vi "DSF.Shared.Constants.Library Name.Engine.vi"() -> (3 "Engine Library Name":string)   [LabVIEW 2017, in "DSF.Engine.lvlib"]
uses:
  DSF.Engine.lvlib
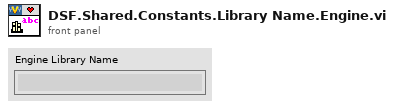
[diagram p1: front panel]
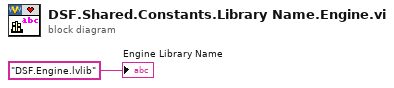
[diagram p0: block diagram]
diagram:
  "Engine Library Name" <- "DSF.Engine.lvlib" ("Library Name")
